vi "Action for NN to real action.vi"(11 "Action":i32) -> (3 "Real action":i16)   [LabVIEW 2013]
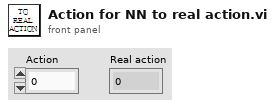
[diagram p1: front panel]
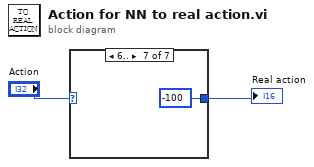
[diagram p0: block diagram]
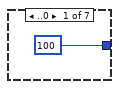
[diagram p2: hidden frame]
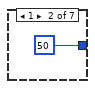
[diagram p3: hidden frame]
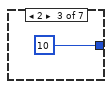
[diagram p4: hidden frame]
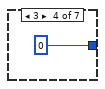
[diagram p5: hidden frame]
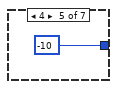
[diagram p6: hidden frame]
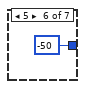
[diagram p7: hidden frame]
diagram:
  n1 = case shown="6.." "Action" {
    tunnel: [i16 100 ("new element/subarray") i16 50 ("new element/subarray") i16 10 ("new element/subarray") i16 0 ("new element/subarray") i16 -10 ("new element/subarray") i16 -50 ("new element/subarray") i16 -100 ("new element/subarray")] -> w1
    frame ..0 {
    }
    frame 1 {
    }
    frame 2 {
    }
    frame 3 {
    }
    frame 4 {
    }
    frame 5 {
    }
    frame 6.. {
    }
  }
  "Real action" <- w1
